vi "FunctionGeneratorMatrix_Add_Value.vi"(9 "Y Value":T1, 10 "X Value":dbl, 11 "in FUNC_GEN_MATRIX":T2) -> (0 "Error":bool, 3 "out FUNC_GEN_MATRIX":T2)   [LabVIEW 2019, in "Trajectory_Library.lvlib"]
doc: "Insert new X, Y pair into an existing Function Generator Matrix data cluster.\n\nInputs:\n - Input Funct Gen Matrix -- Data cluster\n - X Value -- New X value\n - Y Value -- New Y matrix\n\nOutputs:\n - Function Generator Matrix -- Updated data cluster\n - Error -- Set true if an error occured. This is set when the size of the Y matrix does not match the definiton of this function generator."
uses:
  Trajectory_Library.lvlib
  TypeDef/FUNCTION_GENERATOR_MATRIX.ctl
  <vilib>/Analysis/Matrix/Datatypes/RealMatrix.ctl
  <vilib>/gmath/NI_Gmath.lvlib
  <vilib>/Analysis/Matrix/NI_Matrix.lvlib
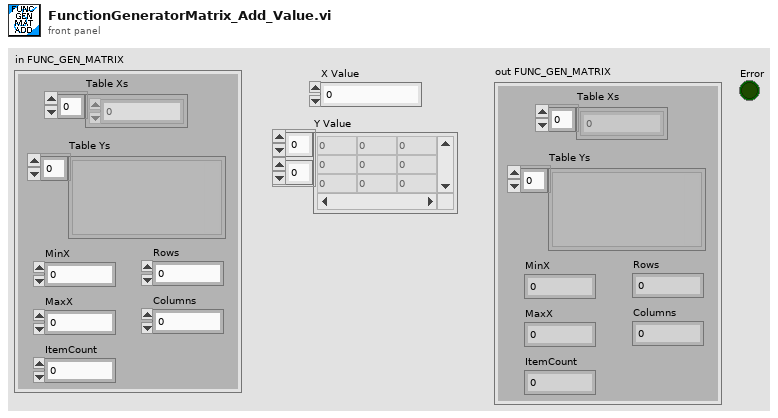
[diagram p1: front panel]
types:
  T1 = typedef "NI_Matrix.lvlib/RealMatrix.ctl" = dbl[][]
  T2 = typedef "Trajectory_Library.lvlib/FUNCTION_GENERATOR_MATRIX.ctl" = cluster{"Table Xs":dbl[], "Table Ys":variant[], "MinX":dbl, "MaxX":dbl, "ItemCount":i32, "Rows":i32, "Columns":i32}
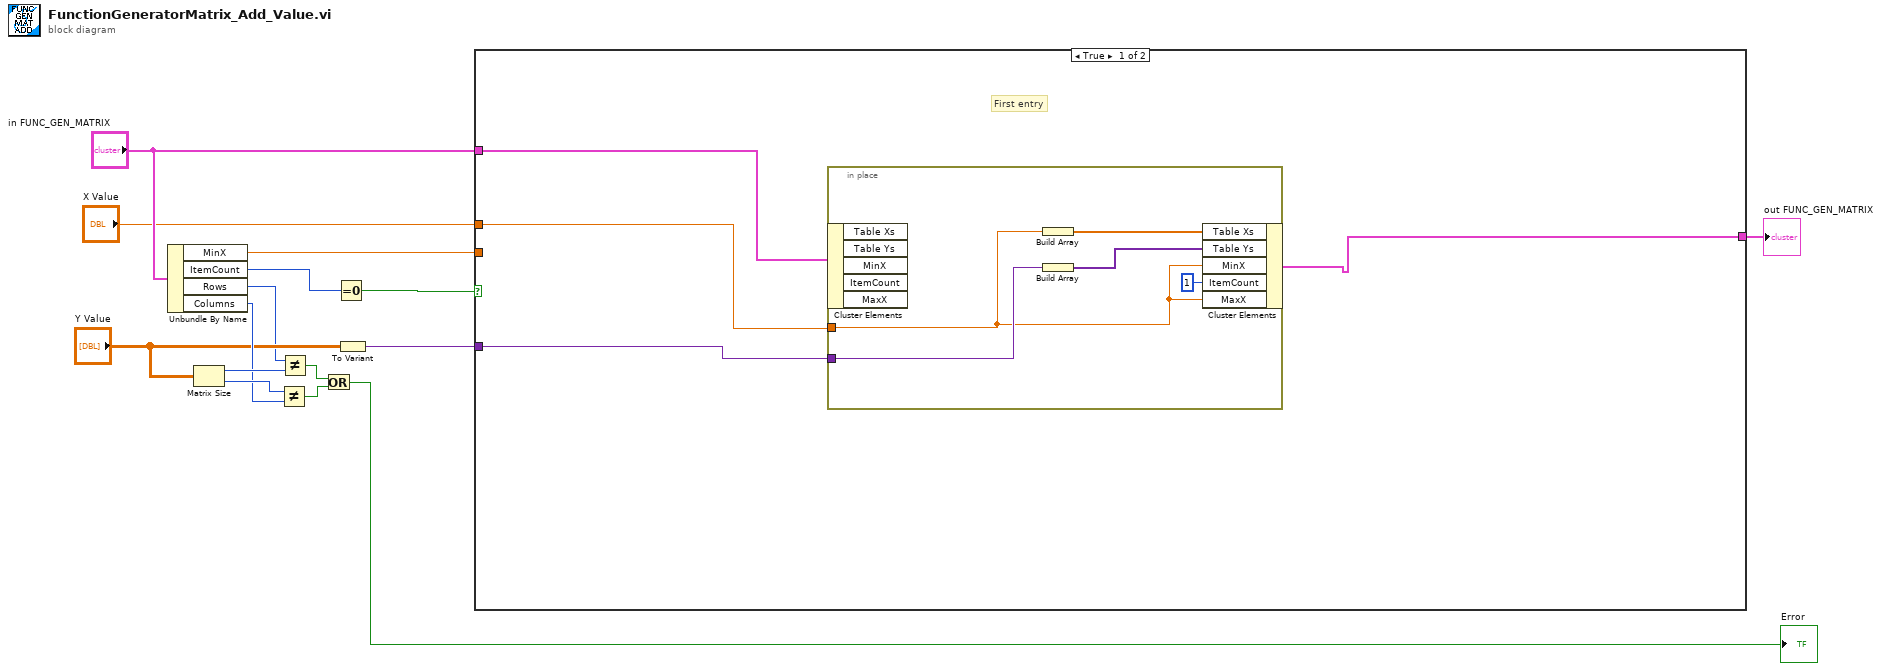
[diagram p0: block diagram]
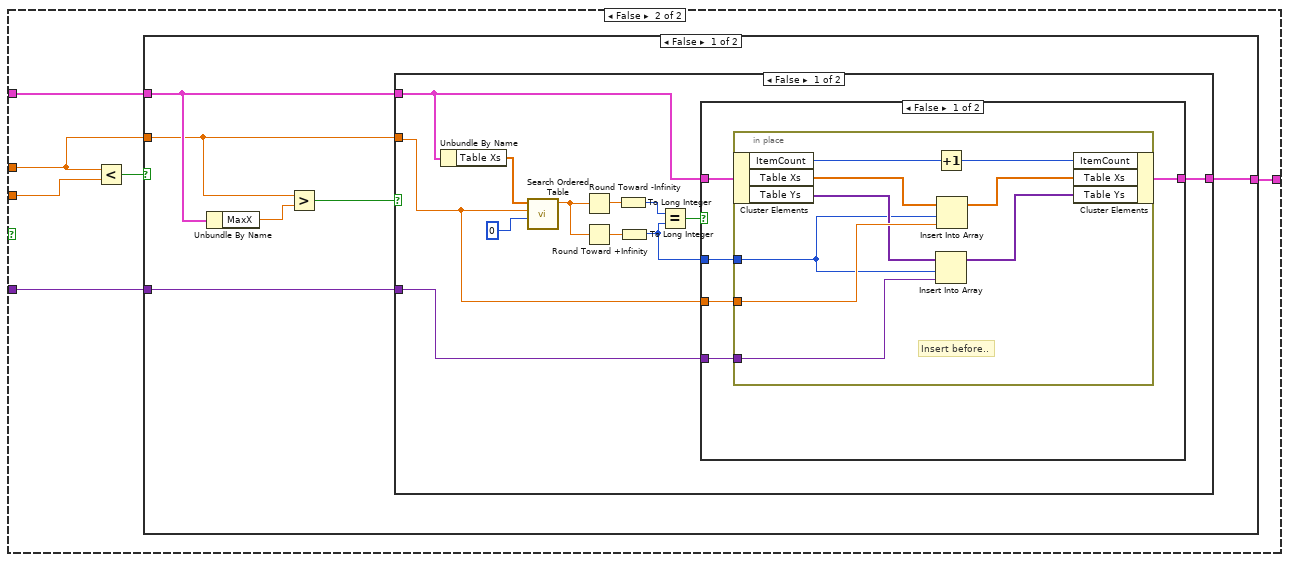
[diagram p2: hidden frame]
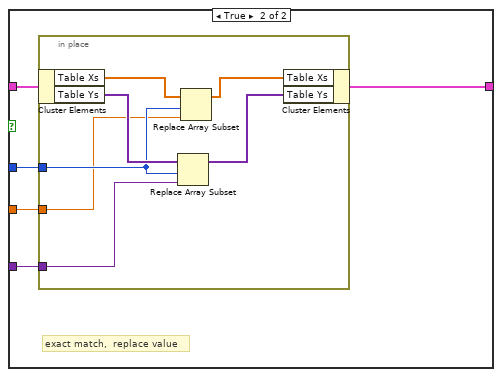
[diagram p3: hidden frame]
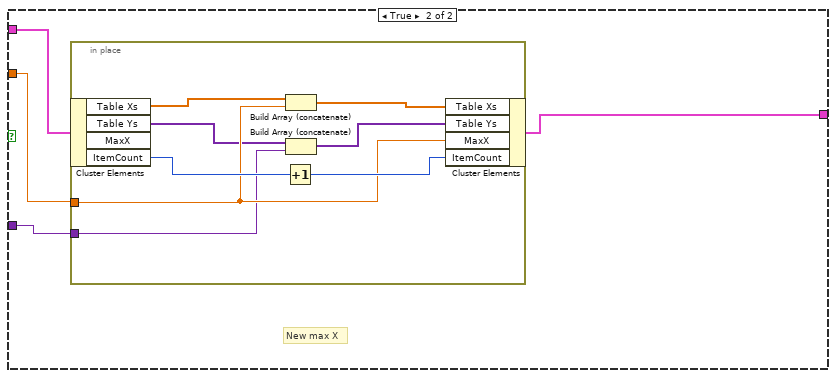
[diagram p4: hidden frame]
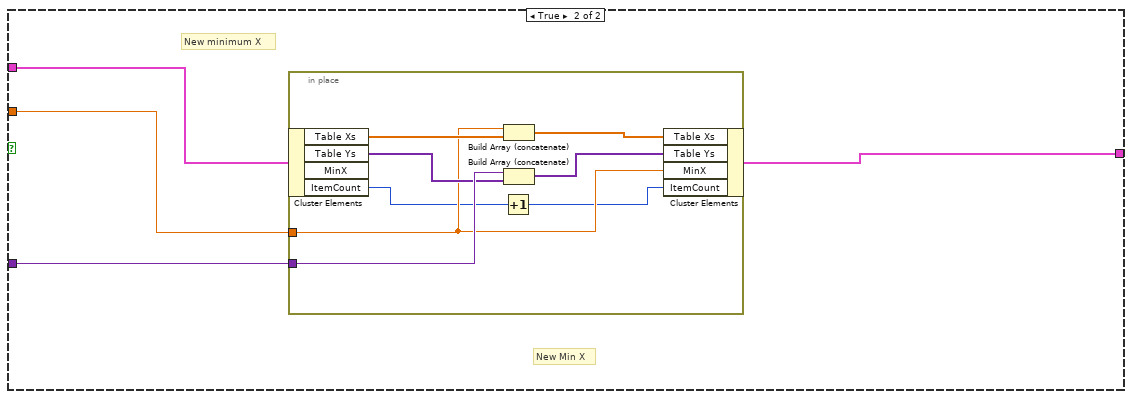
[diagram p5: hidden frame]
diagram:
  n1 = Unbundle By Name("in FUNC_GEN_MATRIX") -> ("MinX"=w15:dbl, "ItemCount"=w2:i32, "Rows"=w3:i32, "Columns"=w9:i32)
  n2 = Matrix Size(0:"Y Value") -> (1:w11:i32, 2:w10:i32)
  n3 = Not Equal?(x=w10, y=w9) -> (x != y?=w7:bool)
  n4 = Not Equal?(x=w3, y=w11) -> (x != y?=w8:bool)
  n5 = Or(x=w8, y=w7) -> (x .or. y?=→"Error":bool)
  n6 = Equal To 0?(x=w2) -> (x = 0?=w1:bool)
  n7 = To Variant(anything="Y Value") -> (Variant=w4:variant)
  n8 = case shown="True" w1 {
    tunnel: w15 -> [_ w30]
    tunnel: "in FUNC_GEN_MATRIX" -> [w19 w28]
    tunnel: "X Value" -> [w18 w27]
    tunnel: [w16 w26] -> w12
    tunnel: w4 -> [w17 w25]
    frame True {
      # "First entry"
      n9 = in-place {
        in-place-border: w18 -> [w21]
        in-place-border: w17 -> [w24]
        n10 = in-place-cluster #1(w19) -> ()  [unwired: 5 out]
        n11 = Build Array(w21) -> (w23:dbl[])
        n12 = Build Array(w24) -> (w22:variant[])
        n13 = in-place-cluster #1("Table Xs"=w23, "Table Ys"=w22, "MinX"=w21, "ItemCount"=1, "MaxX"=w21) -> (w16:T2)
      }
    }
    frame False {
      n14 = Less?(x=w27, y=w30) -> (x < y?=w29:bool)
      n15 = case shown="False" w29 {
        tunnel: w28 -> [w35 w90]
        tunnel: w27 -> [w33 w89]
        tunnel: w25 -> [w32 w88]
        tunnel: [w34 w87] -> w26
        frame False {
          n16 = Unbundle By Name(w35) -> ("MaxX"=w36:dbl)
          n17 = Greater?(x=w33, y=w36) -> (0:w31:bool)
          n18 = case shown="False" w31 {
            tunnel: w35 -> [w41 w78]
            tunnel: [w37 w77] -> w34
            tunnel: w33 -> [w39 w76]
            tunnel: w32 -> [w38 w75]
            frame False {
              n19 = Unbundle By Name(w41) -> ("Table Xs"=w47:dbl[])
              n20 = call <vilib>:"Search Ordered Table.vi"("starting index"=0, "x value"=w39, "ordered x array"=w47) -> ("fractional index"=w46:dbl)  [unwired: 8 in]
              n21 = Round Toward -Infinity(1:w46) -> (0:w44:dbl)
              n22 = Round Toward +Infinity(x=w46) -> (ceil(x): smallest int >= x=w45:dbl)
              n23 = To Long Integer(number=w44) -> (32bit integer=w43:i32)
              n24 = To Long Integer(number=w45) -> (32bit integer=w40:i32)
              n25 = Equal?(x=w43, y=w40) -> (x = y?=w42:bool)
              n26 = case shown="False" w42 {
                tunnel: w41 -> [w50 w67]
                tunnel: w40 -> [w53 w66]
                tunnel: w39 -> [w52 w65]
                tunnel: w38 -> [w51 w64]
                tunnel: [w49 w63] -> w37
                frame False {
                  n27 = in-place {
                    in-place-border: w53 -> [w57]
                    in-place-border: w52 -> [w59]
                    in-place-border: w51 -> [w56]
                    # "Insert before.."
                    n28 = in-place-cluster #2(w50) -> ("ItemCount"=w62:i32, "Table Xs"=w60:dbl[], "Table Ys"=w58:variant[])
                    n29 = Increment(x=w62) -> (x+1=w61:i32)
                    n30 = Insert Into Array(array=w58, index=w57, new element=w56) -> (w54:variant[])
                    n31 = Insert Into Array(array=w60, index=w57, new element=w59) -> (w55:dbl[])
                    n32 = in-place-cluster #2("ItemCount"=w61, "Table Xs"=w55, "Table Ys"=w54) -> (w49:T2)
                  }
                }
                frame True {
                  # "exact match,  replace value"
                  n33 = in-place {
                    in-place-border: w66 -> [w72]
                    in-place-border: w65 -> [w71]
                    in-place-border: w64 -> [w70]
                    n34 = in-place-cluster #3(w67) -> ("Table Xs"=w74:dbl[], "Table Ys"=w73:variant[])
                    n35 = Replace Array Subset(array=w73, new element=w70, index=w72) -> (w68:variant[])
                    n36 = Replace Array Subset(array=w74, new element=w71, index=w72) -> (w69:dbl[])
                    n37 = in-place-cluster #3("Table Xs"=w69, "Table Ys"=w68) -> (w63:T2)
                  }
                }
              }
            }
            frame True {
              # "New max X"
              n38 = in-place {
                in-place-border: w76 -> [w82]
                in-place-border: w75 -> [w79]
                n39 = in-place-cluster #4(w78) -> ("Table Xs"=w81:dbl[], "Table Ys"=w80:variant[], "ItemCount"=w84:i32)  [unwired: 1 out]
                n40 = Increment(x=w84) -> (x+1=w83:i32)
                n41 = Build Array (concatenate)(w81, w82) -> (w86:dbl[])
                n42 = Build Array (concatenate)(w80, w79) -> (w85:variant[])
                n43 = in-place-cluster #4("Table Xs"=w86, "Table Ys"=w85, "MaxX"=w82, "ItemCount"=w83) -> (w77:T2)
              }
            }
          }
        }
        frame True {
          # "New Min X"
          # "New minimum X"
          n44 = in-place {
            in-place-border: w89 -> [w93]
            in-place-border: w88 -> [w98]
            n45 = in-place-cluster #5(w90) -> ("Table Xs"=w97:dbl[], "Table Ys"=w94:variant[], "ItemCount"=w92:i32)  [unwired: 1 out]
            n46 = Increment(x=w92) -> (x+1=w91:i32)
            n47 = Build Array (concatenate)(w93, w97) -> (w96:dbl[])
            n48 = Build Array (concatenate)(w98, w94) -> (w95:variant[])
            n49 = in-place-cluster #5("Table Xs"=w96, "Table Ys"=w95, "MinX"=w93, "ItemCount"=w91) -> (w87:T2)
          }
        }
      }
    }
  }
  "out FUNC_GEN_MATRIX" <- w12
